vi "CH1_Manual_range_select.vi"(9 "CH1":u8(knob) scale=0.0..3.0, 10 "EN":bool, 11 "Select COM port":refnum<visa-resource-name>="COM3") -> (2 "CH1 IN2 R":string)   [LabVIEW 2012]
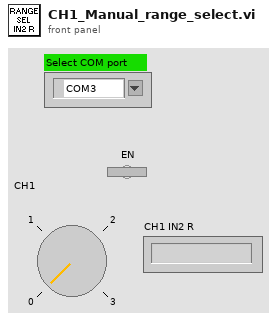
[diagram p1: front panel]
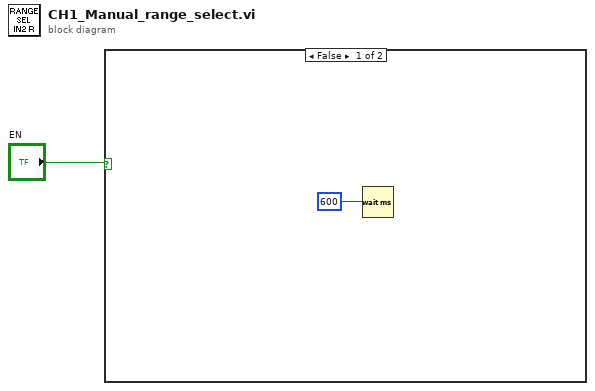
[diagram p0: block diagram]
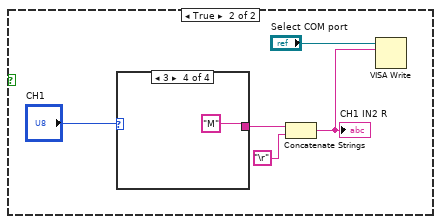
[diagram p2: hidden frame]
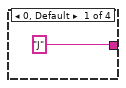
[diagram p3: hidden frame]
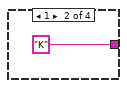
[diagram p4: hidden frame]
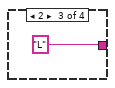
[diagram p5: hidden frame]
diagram:
  n1 = case shown="False" "EN" {
    frame False {
      n2 = Wait (ms)(milliseconds to wait=600) -> ()  [unwired: 1 out]
    }
    frame True {
      n3 = case shown="3" "CH1" {
        tunnel: ["J" "K" "L" "M"] -> w6
        frame 0, Default {
        }
        frame 1 {
        }
        frame 2 {
        }
        frame 3 {
        }
      }
      n4 = Concatenate Strings(w6, "\r") -> (w3:string)
      "CH1 IN2 R" <- w3
      n5 = VISA Write(VISA resource name="Select COM port", write buffer=w3) -> ()  [unwired: 1 in, 3 out]
    }
  }
